vi "Google Earth - Version info.vi"(8 "error in":errorcluster, 11 "Refnum In":refnum<k7>) -> (0 "error out":errorcluster, 1 "VersionMinor":i32, 2 "VersionMajor":i32, 3 "Refnum Out":refnum<k7>, 4 "VersionBuild":i32, 5 "VersionAppType":i32(ring) items=["EnterpriseClientGE"=0, "ProGE"=1, "PlusGE"=2, "FreeGE"=5, "UnknownGE"=255])   [LabVIEW 2015]
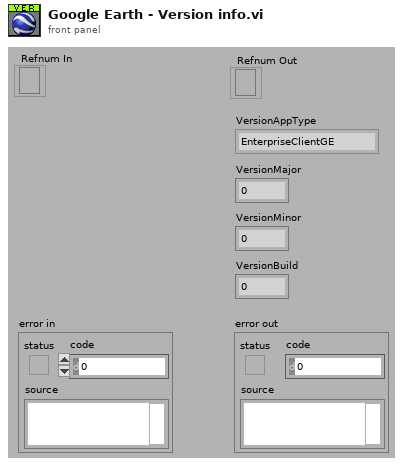
[diagram p1: front panel]
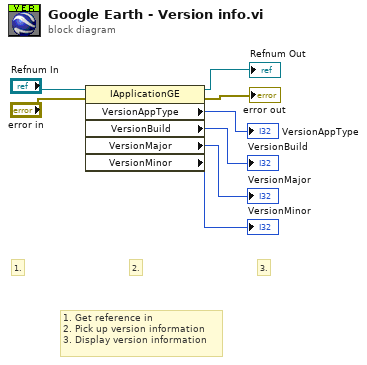
[diagram p0: block diagram]
diagram:
  # "1. Get reference in\n2. Pick up version information\n3. Display version information"
  # "3."
  # "2."
  # "1."
  n1 = property class="IApplicationGE"(reference="Refnum In", error in="error in") -> (reference out=→"Refnum Out":refnum<k7>, error out=→"error out":errorcluster, "VersionAppType"=→"VersionAppType":i32, "VersionBuild"=→"VersionBuild":i32, "VersionMajor"=→"VersionMajor":i32, "VersionMinor"=→"VersionMinor":i32)
